vi "Hello_Oleg.vi"   [LabVIEW 2015]
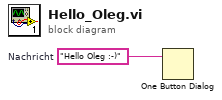
[diagram p0: block diagram]
diagram:
  w1 = "Hello Oleg :-)"  # Nachricht
  n1 = One Button Dialog(message=w1) -> ()  [unwired: 1 in, 1 out]
